vi "write pre and post build refs .vi"(10 "pre and post build refs":refnum<vi>[](array[refnum]), 11 "Builders in":refnum<class "Builder.lvclass">) -> (3 "Builders out":refnum<class "Builder.lvclass">)   [LabVIEW 2024, in "Builder.lvclass"]
uses:
  Builder.lvclass
  Builder.lvclass/Builder.ctl
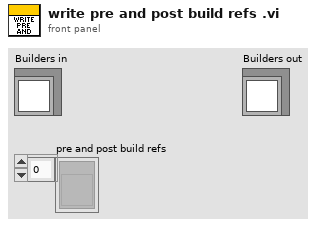
[diagram p1: front panel]
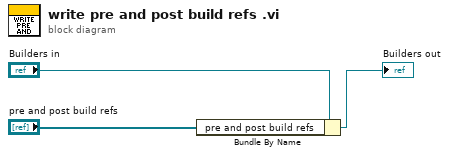
[diagram p0: block diagram]
diagram:
  n1 = Bundle By Name(cluster="Builders in", "pre and post build refs"="pre and post build refs") -> (→"Builders out":refnum<class "Builder.lvclass">)
